vi "err_handler.vi"(11 "error in (no error)":errorcluster) -> ()   [LabVIEW 2016]
uses:
  <vilib>/Utility/error.llb/DialogType.ctl
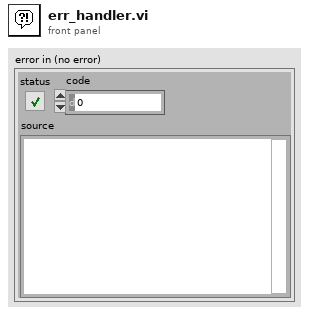
[diagram p1: front panel]
types:
  T1 = typedef "DialogType.ctl" = u16
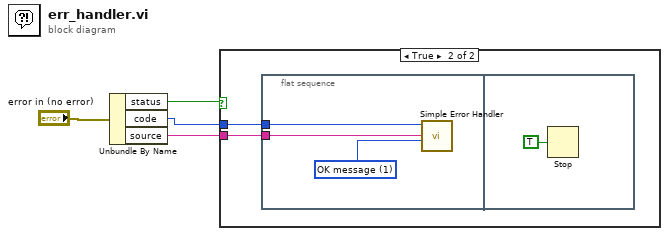
[diagram p0: block diagram]
diagram:
  n1 = Unbundle By Name("error in (no error)") -> ("status"=w3:bool, "code"=w2:i32, "source"=w1:string)
  n2 = case shown="True" w3 {
    tunnel: w2 -> [_ w6]
    tunnel: w1 -> [_ w5]
    frame False {
    }
    frame True {
      n3 = flat-sequence {
        tunnel: w6 -> [w8]
        tunnel: w5 -> [w7]
        frame #0 {
          w9 = T1 1 items=["no dialog", "OK message", "continue or stop message", "OK message + warnings", "continue/stop + warnings"] ("type of dialog (OK msg:1)")
          n4 = call <vilib>:"Simple Error Handler.vi"("error code (no error:0)"=w8, "error source (\" \")"=w7, "type of dialog (OK msg:1)"=w9) -> ()  [unwired: 2 in, 5 out]
        }
        frame #1 {
          n5 = Stop(stop? (T)=TRUE) -> ()
        }
      }
    }
  }
